vi "scan test data.vi"(10 "error in":errorcluster, 11 "file path in":path) -> (1 "file path out":path, 2 "error out":errorcluster, 3 "Array":u8[][](array[numeric]) format="%x")   [LabVIEW 2017, in "SPELS test.lvlib"]
uses:
  SPELS test.lvlib
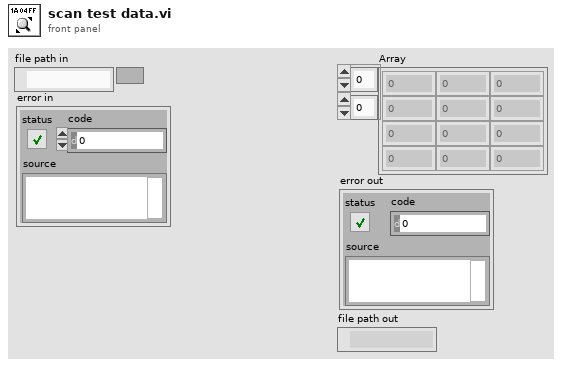
[diagram p1: front panel]
types:
  T1 = enum16{"open", "replace", "create", "open or create", "replace or create", "replace or create with confirmation"}
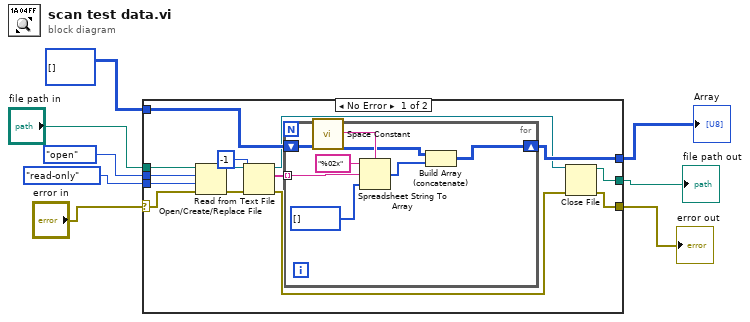
[diagram p0: block diagram]
diagram:
  n1 = case shown="No Error" "error in" {
    selector: "error in" -> [w17 w31]
    tunnel: "file path in" -> [w22 w30]
    tunnel: T1."open" ("operation (0:open)") -> [w21 _]
    tunnel: enum16{"read/write", "read-only", "write-only"}."read-only" ("access (0:read/write)") -> [w20 _]
    tunnel: [w14 w32] -> w4
    tunnel: u8[][] [] -> [w13 w32]
    tunnel: [w9 w31] -> w2
    tunnel: [w12 w30] -> w1
    frame No Error {
      n2 = Open/Create/Replace File(file path (use dialog)=w22, error in=w17, operation (0:open)=w21, access (0:read/write)=w20) -> (refnum out=w19:refnum<file>, error out=w18:errorcluster)  [unwired: 2 in, 1 out]
      n3 = Read from Text File(file (use dialog)=w19, count=-1, error in=w18) -> (refnum out=w11:refnum<file>, text=w15:string[], error out=w10:errorcluster)  [unwired: 1 in, 1 out]
      n4 = for {
        tunnel: w15 -> [w29] mode=indexing
        shift-right: [w23] -> w14
        shift-left: w13 -> [w24]
        n5 = call <vilib>:"Space Constant.vi"() -> ("String"=w27:string)
        n6 = Spreadsheet String To Array(delimiter (Tab)=w27, format string="%02x", spreadsheet string=w29, array type (2D Dbl)=u8[] []) -> (array=w25:u8[])
        n7 = Build Array (concatenate)(w24, w25) -> (w23:u8[][])
      }
      n8 = Close File(refnum=w11, error in=w10) -> (path=w12:path, error out=w9:errorcluster)
    }
    frame Error {
    }
  }
  "Array" <- w4
  "error out" <- w2
  "file path out" <- w1
